vi "Fire USER EVents.vi"() -> ()   [LabVIEW 2019]
panel:
  in  "stop":bool
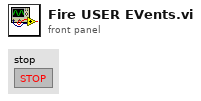
[diagram p1: front panel]
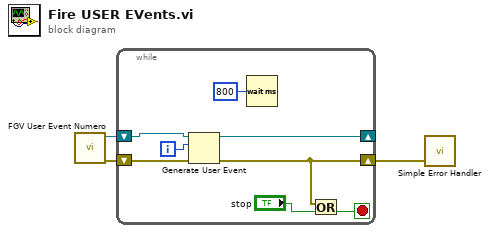
[diagram p0: block diagram]
diagram:
  n1 = call "FGV User Event Numero.vi"() -> ("error out"=w3:errorcluster, "User Event Numero"=w2:refnum<user-event>)  [unwired: 10 in]
  n2 = while {
    shift-right: [w4] -> w1
    shift-left: w3 -> [w11]
    shift-right: [w10] -> _
    shift-left: w2 -> [w9]
    i -> [w8]
    stop <- w5 stop-if-true
    n3 = Generate User Event(user event=w9, event data cluster=w8, error in=w11) -> (user event out=w10:refnum<user-event>, error out=w4:errorcluster)  [unwired: 1 in]
    n4 = Wait (ms)(milliseconds to wait=u32 800) -> ()  [unwired: 1 out]
    n5 = Or(x=w4, y="stop") -> (x .or. y?=w5:bool)
  }
  n6 = call <vilib>:"Simple Error Handler.vi"("error in (no error)"=w1) -> ()  [unwired: 4 in, 5 out]
